vi "Get Next Question.vi"(10 "Candidate_ID":string, 11 "Candidates":T1[](array[typedef])) -> (3 "Candidates out":T1[](array[typedef]))   [LabVIEW 2014, in "Coding Platform.lvlib"]
uses:
  Coding Platform.lvlib
  Typedefs/Candidate.ctl
  Typedefs/Candidate State.ctl
  Typedefs/Answer Info.ctl
  Typedefs/Answer State.ctl
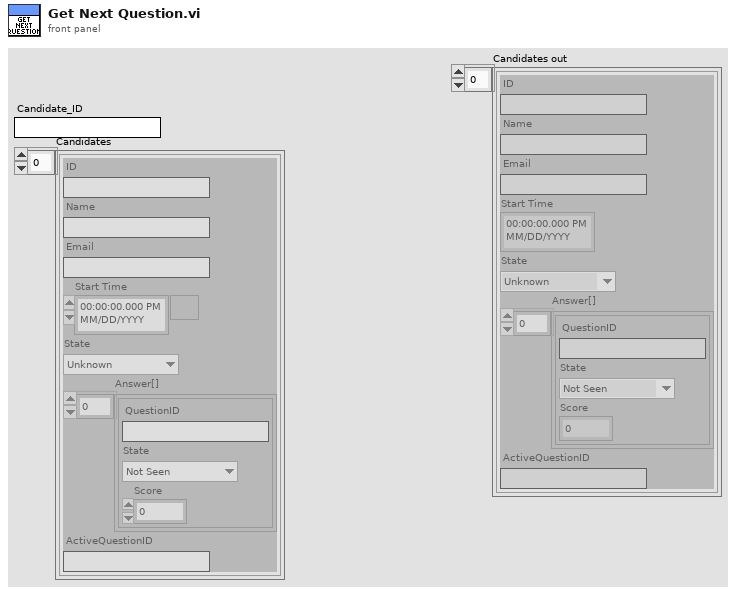
[diagram p1: front panel]
types:
  T1 = typedef "Coding Platform.lvlib/Candidate.ctl" = cluster{"ID":string, "Name":string, "Email":string, "Start Time":timestamp, "State":T2, "Answer[]":T3[], "ActiveQuestionID":string}
  T2 = typedef "Coding Platform.lvlib/Candidate State.ctl" = enum16{"Unknown", "LoggedIn", "In Test", "Completed Test"}
  T3 = typedef "Coding Platform.lvlib/Answer Info.ctl" = cluster{"QuestionID":string, "State":T4, "Score":u64}
  T4 = typedef "Coding Platform.lvlib/Answer State.ctl" = enum16{"Not Seen", "In Progress", "Completed"}
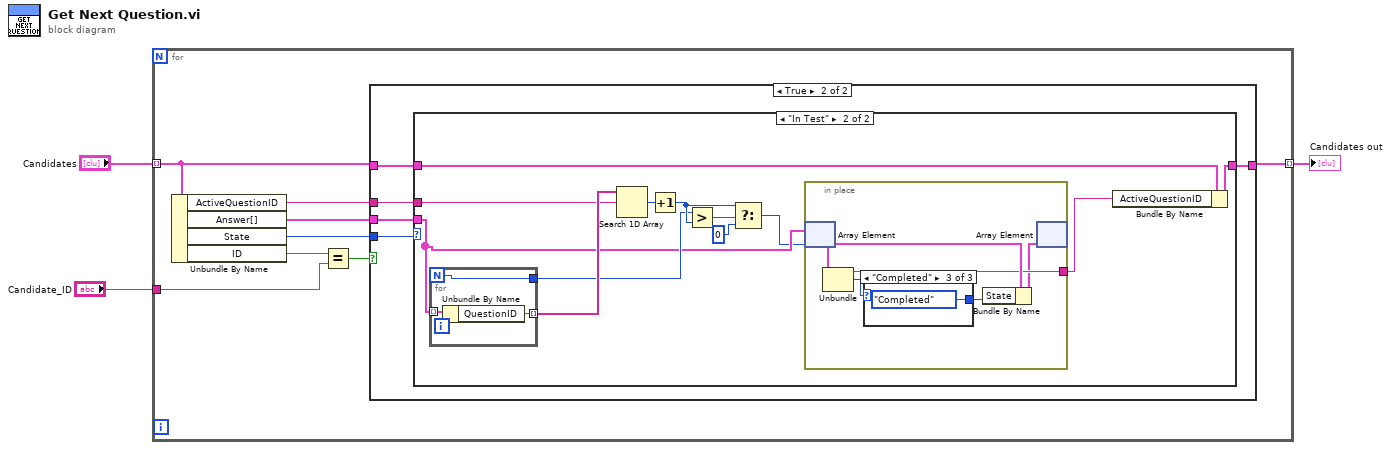
[diagram p0: block diagram]
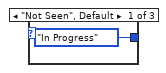
[diagram p4: hidden frame]
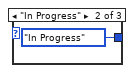
[diagram p5: hidden frame]
diagram:
  n1 = for {
    tunnel: "Candidate_ID" -> [w10]
    tunnel: [w7] -> w1 mode=indexing
    tunnel: "Candidates" -> [w6] mode=indexing
    n2 = Unbundle By Name(w6) -> ("ActiveQuestionID"=w4:string, "Answer[]"=w5:T3[], "State"=w8:T2, "ID"=w11:string)
    n3 = Equal?(x=w11, y=w10) -> (x = y?=w9:bool)
    n4 = case shown="True" w9 {
      tunnel: w8 -> [_ w14]
      tunnel: [w12 w15] -> w7
      tunnel: w6 -> [w12 w17]
      tunnel: w5 -> [_ w16]
      tunnel: w4 -> [_ w13]
      frame False {
      }
      frame True {
        n5 = case shown="\"In Test\"" w14 {
          tunnel: w17 -> [w18 w30]
          tunnel: w16 -> [_ w22]
          tunnel: [w18 w20] -> w15
          tunnel: w13 -> [_ w25]
          frame "Unknown", Default {
          }
          frame "In Test" {
            n6 = for {
              N -> [w39]
              tunnel: w22 -> [w41] mode=indexing
              tunnel: [w40] -> w26 mode=indexing
              tunnel: [w39] -> w24
              n7 = Unbundle By Name(w41) -> ("QuestionID"=w40:string)
            }
            n8 = Search 1D Array(1D array=w26, element=w25) -> (index of element=w23:i32)  [unwired: 1 in]
            n9 = Increment(x=w23) -> (x+1=w27:i32)
            n10 = Greater?(x=w24, y=w27) -> (0:w29:bool)
            n11 = Select(t=w27, s=w29, f=0) -> (s? t:f=w21:i32)
            n12 = in-place {
              in-place-border: [w34] -> w19
              n13 = in-place-array #1(w22, w21) -> (w35:T3)
              n14 = Unbundle(w35) -> ("QuestionID"=w34:string, "State"=w31:T4)  [unwired: 1 out]
              n15 = case shown="\"Completed\"" w31 {
                tunnel: [Answer_State."In Progress" ("State") Answer_State."In Progress" ("State") Answer_State."Completed" ("State")] -> w32
                frame "Not Seen", Default {
                }
                frame "In Progress" {
                }
                frame "Completed" {
                }
              }
              n16 = Bundle By Name(cluster=w35, "State"=w32) -> (w33:T3)
              n17 = in-place-array #1(w33) -> ()  [unwired: 2 out]
            }
            n18 = Bundle By Name(cluster=w30, "ActiveQuestionID"=w19) -> (w20:T1)
          }
        }
      }
    }
  }
  "Candidates out" <- w1
